vi "ReadChannel.vi"(8 "error in (no error)":errorcluster, 11 "Television in":refnum<class "Television.lvclass">) -> (0 "error out":errorcluster, 2 "Channel":i32, 3 "Television out":refnum<class "Television.lvclass">)   [LabVIEW 2013, in "Television.lvclass"]
uses:
  Television.lvclass
  Television.lvclass/Television.ctl
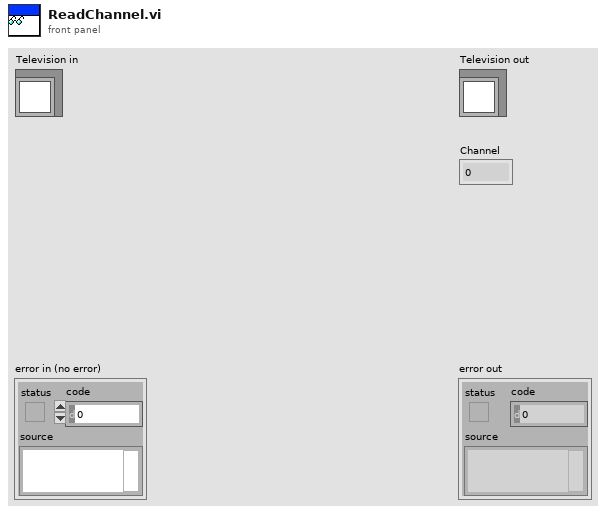
[diagram p1: front panel]
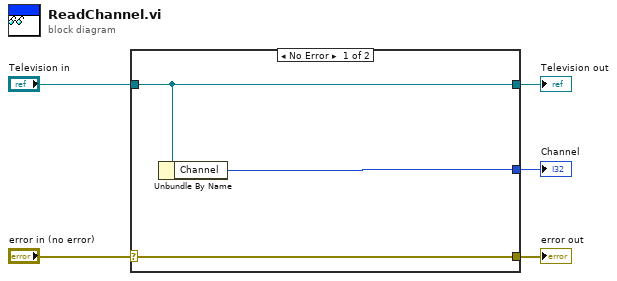
[diagram p0: block diagram]
diagram:
  n1 = case shown="No Error" "error in (no error)" {
    selector: "error in (no error)" -> [w8 w9]
    tunnel: [w8 w9] -> w4
    tunnel: [w7 w10] -> w2
    tunnel: "Television in" -> [w7 w10]
    tunnel: [w6 _] -> w1
    frame No Error {
      n2 = Unbundle By Name(w7) -> ("Channel"=w6:i32)
    }
    frame Error {
    }
  }
  "error out" <- w4
  "Television out" <- w2
  "Channel" <- w1
